vi "save_camera_raw.vi"(7 "Array of Images":T1[][](array[typedef]), 8 "error in (no error)":errorcluster, 10 "XYZC iteration string":string, 11 "Data Files Path":path=path "C:/Users/QCC/Documents/Cesium_project/LabVIEW Projects/data/2011_03_02") -> (0 "error out":errorcluster)   [LabVIEW 2011]
uses:
  <vilib>/vision/Image Controls.llb/IMAQ Image.ctl
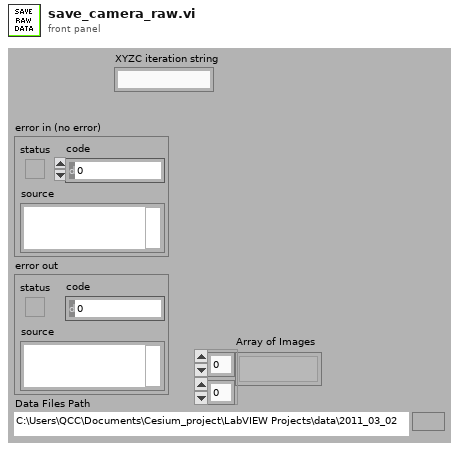
[diagram p1: front panel]
types:
  T1 = typedef "IMAQ Image.ctl" = refnum<image>
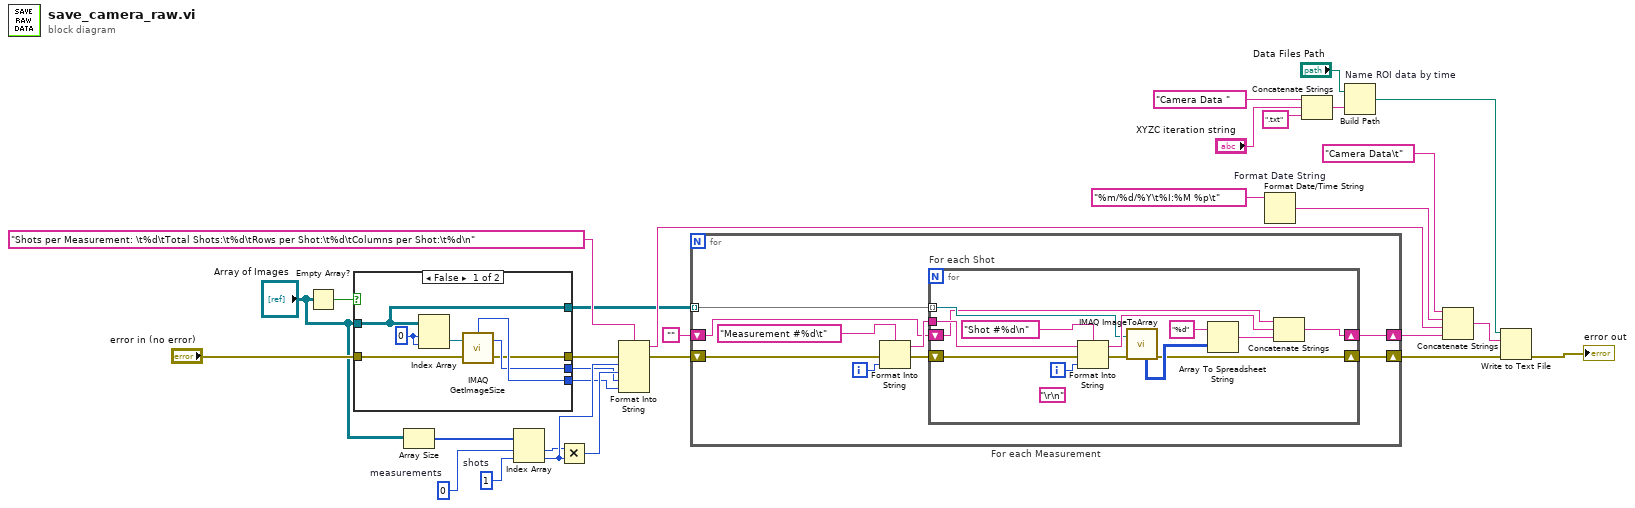
[diagram p0: block diagram]
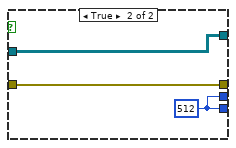
[diagram p2: hidden frame]
diagram:
  w23 = 1  # shots
  w24 = 0  # measurements
  n1 = Empty Array?(array="Array of Images") -> (empty?=w7:bool)
  n2 = case shown="False" w7 {
    tunnel: [w33 w40] -> w6
    tunnel: [w34 w40] -> w5
    tunnel: "Array of Images" -> [w31 w38]
    tunnel: "error in (no error)" -> [w35 w39]
    tunnel: [w32 w39] -> w3
    tunnel: [w31 w38] -> w1
    frame False {
      w37 = 0 ("index (row)")
      n3 = Index Array(array=w31, index (row)=w37, index (col)=w37) -> (element=w36:T1)
      n4 = call "IMAQ GetImageSize"("Image"=w36, "error in (no error)"=w35) -> ("Y Resolution"=w33:i32, "X Resolution"=w34:i32, "error out"=w32:errorcluster)  [unwired: 2 in]
    }
    frame True {
      w40 = 512
    }
  }
  n5 = Array Size(array="Array of Images") -> (size(s)=w25:i32[])
  n6 = Index Array(array=w25, index #1=w24, index #2=w23) -> (element #1=w19:i32, element #2=w20:i32)
  n7 = Multiply(x=w19, y=w20) -> (x*y=w18:i32)
  n8 = Format Into String(format string="Shots per Measurement: \t%d\tTotal Shots:\t%d\tRows per Shot:\t%d\tColumns per Shot:\t%d\n", error in=w3, w20, w18, w6, w5) -> (resulting string=w14:string, error out=w11:errorcluster)  [unwired: 1 in]
  n9 = for "For each Measurement" {
    tunnel: w1 -> [w45] mode=indexing
    shift-right: [w42] -> w17
    shift-left: w11 -> [w43]
    shift-right: [w49] -> w15
    shift-left: "" -> [w41]
    i -> [w47]
    n10 = Format Into String(format string="Measurement #%d\t", error in=w43, w47) -> (resulting string=w46:string, error out=w44:errorcluster)  [unwired: 1 in]
    n11 = for "For each Shot" {
      tunnel: w46 -> [w60]
      tunnel: w45 -> [w57] mode=indexing
      shift-right: [w51] -> w42
      shift-left: w44 -> [w52]
      shift-right: [w62] -> w49
      shift-left: w41 -> [w50]
      i -> [w61]
      (unwired) "\r\n"
      n12 = Format Into String(format string="Shot #%d\n", initial string=w60, error in=w52, w61) -> (resulting string=w58:string, error out=w53:errorcluster)
      n13 = call "IMAQ ImageToArray"("error in (no error)"=w53, "Image"=w57) -> ("Image Pixels (U16)"=w56:u16[][], "error out"=w51:errorcluster)  [unwired: 2 in, 3 out]
      n14 = Array To Spreadsheet String(array=w56, 3:"%d" ("format string")) -> (spreadsheet string=w54:string)  [unwired: 1 in]
      n15 = Concatenate Strings(w50, w58, w54) -> (w62:string)
    }
  }
  n16 = Format Date/Time String "Format Date String"(time format string (%c)="%m/%d/%Y\t%I:%M %p\t") -> (date/time string=w12:string)  [unwired: 2 in]
  n17 = Concatenate Strings("Camera Data ", "XYZC iteration string", ".txt" ("string")) -> (w28:string)
  n18 = Build Path "Name ROI data by time"(base path="Data Files Path", name or relative path=w28) -> (appended path=w29:path)
  n19 = Concatenate Strings("Camera Data\t", w12, w14, w15) -> (w10:string)
  n20 = Write to Text File(file (use dialog)=w29, text=w10, error in=w17) -> (error out=→"error out":errorcluster)  [unwired: 1 in, 2 out]
